vi "FPGA_Clock.vi"(0 "Pause":u8=20, 1 "Data":u32=128, 2 "State":T1) -> ()   [LabVIEW 2015]
uses:
  States.ctl
  <vilib>/rvi/Emulation/niFpgaGetClockAttributes.vi
  <vilib>/rvi/Emulation/niFpgaSctlEmulationGetInTimedLoop.vi
  <vilib>/rvi/Emulation/niFpgaEmulationReportErrorSimple.vi
  <vilib>/rvi/eio/common/nirviEmuTemplateMethod_errors.vi
  <vilib>/rvi/Emulation/niFpgaCriticalErrorInLSC.vi
  <vilib>/eio/EIONode/EIONode.xnode
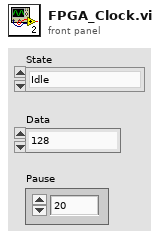
[diagram p1: front panel]
types:
  T1 = typedef "States.ctl" = enum16{"Idle", "CS", "Ready", "Clock High", "Clock Low", "Wait", "Exit"}
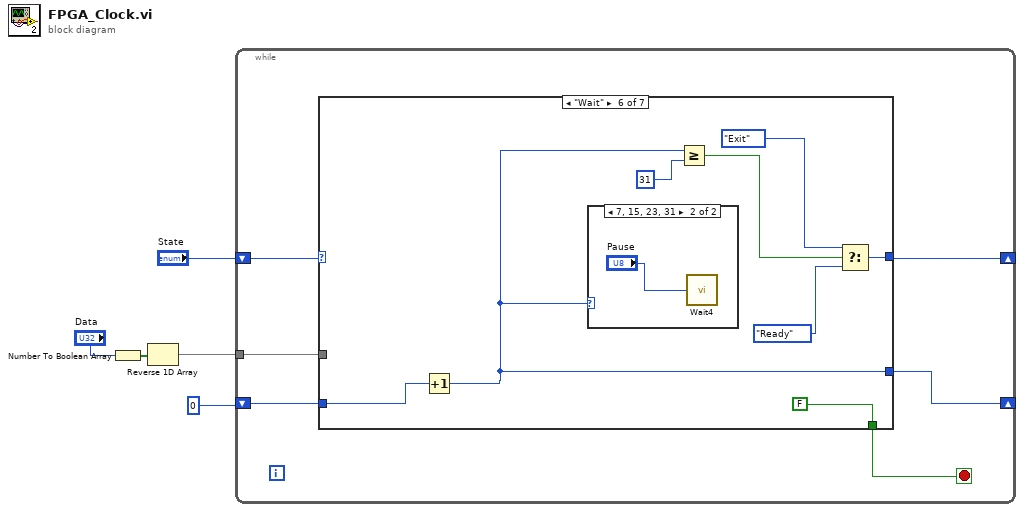
[diagram p0: block diagram]
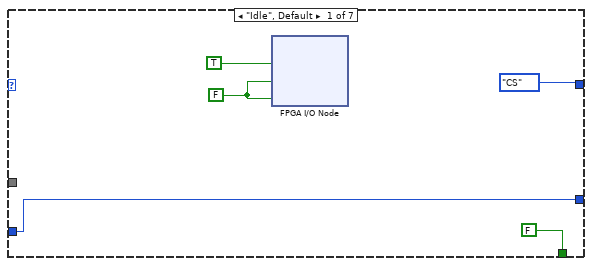
[diagram p2: hidden frame]
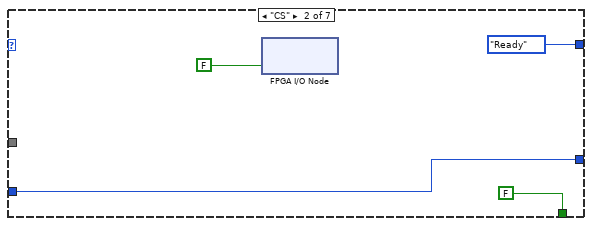
[diagram p3: hidden frame]
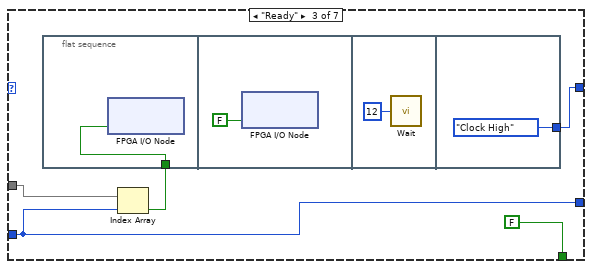
[diagram p4: hidden frame]
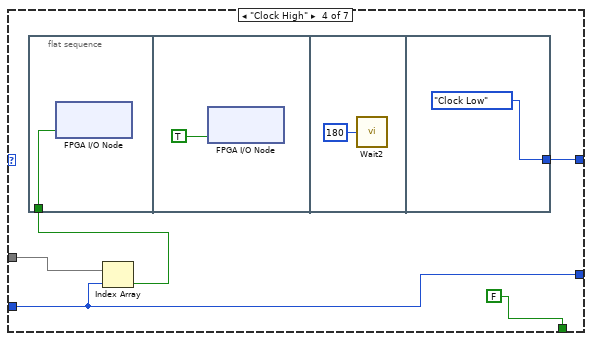
[diagram p5: hidden frame]
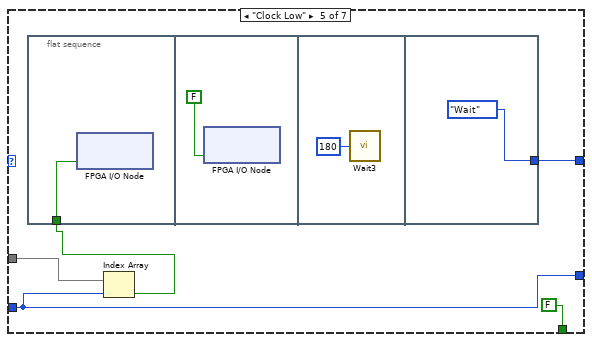
[diagram p6: hidden frame]
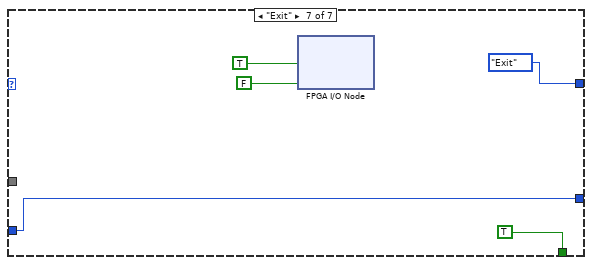
[diagram p8: hidden frame]
diagram:
  n1 = Number To Boolean Array(number="Data") -> (Boolean array=w4:bool[])
  n2 = Reverse 1D Array(array=w4) -> (reversed array=w2:bool[])
  n3 = while {
    shift-right: [w9] -> _
    shift-left: "State" -> [w10]
    tunnel: w2 -> [w8]
    shift-right: [w6] -> _
    shift-left: i16 0 -> [w7]
    stop <- w11 stop-if-true
    n4 = case shown="\"Wait\"" w10 {
      tunnel: [FALSE FALSE FALSE FALSE FALSE FALSE TRUE] -> w11
      tunnel: [States."CS" ("State") States."Ready" ("State") w21 w31 w39 w51 States."Exit" ("State")] -> w9
      tunnel: w8 -> [_ _ w24 w33 w42 _ _]
      tunnel: w7 -> [w13 w17 w23 w32 w41 w49 w58]
      tunnel: [w13 w17 w23 w32 w41 w48 w58] -> w6
      frame "Idle", Default {
        w12 = FALSE
        n5 = xnode "FPGA I/O Node"("CS"=TRUE, "SCLK"=w12, "MOSI"=w12) -> ()  [unwired: 3 in, 3 out]
      }
      frame "CS" {
        n6 = xnode "FPGA I/O Node"("CS"=FALSE) -> ()  [unwired: 1 in, 1 out]
      }
      frame "Ready" {
        n7 = flat-sequence {
          tunnel: w22 -> [w26]
          tunnel: [States."Clock High" ("State")] -> w21
          frame #0 {
            n8 = xnode "FPGA I/O Node"("MOSI"=w26) -> ()  [unwired: 1 in, 1 out]
          }
          frame #1 {
            n9 = xnode "FPGA I/O Node"("SCLK"=FALSE) -> ()  [unwired: 1 in, 1 out]
          }
          frame #2 {
            n10 = call "Wait"("Count(Ticks)"=u8 12) -> ()  [unwired: 1 out]
          }
          frame #3 {
          }
        }
        n11 = Index Array(array=w24, index=w23) -> (element=w22:bool)
      }
      frame "Clock High" {
        n12 = flat-sequence {
          tunnel: w30 -> [w35]
          tunnel: [States."Clock Low" ("State")] -> w31
          frame #0 {
            n13 = xnode "FPGA I/O Node"("MOSI"=w35) -> ()  [unwired: 1 in, 1 out]
          }
          frame #1 {
            n14 = xnode "FPGA I/O Node"("SCLK"=TRUE) -> ()  [unwired: 1 in, 1 out]
          }
          frame #2 {
            n15 = call "Wait2"("Count(Ticks)"=u8 180) -> ()  [unwired: 1 out]
          }
          frame #3 {
          }
        }
        n16 = Index Array(array=w33, index=w32) -> (element=w30:bool)
      }
      frame "Clock Low" {
        n17 = flat-sequence {
          tunnel: w40 -> [w44]
          tunnel: [States."Wait" ("State")] -> w39
          frame #0 {
            n18 = xnode "FPGA I/O Node"("MOSI"=w44) -> ()  [unwired: 1 in, 1 out]
          }
          frame #1 {
            n19 = xnode "FPGA I/O Node"("SCLK"=FALSE) -> ()  [unwired: 1 in, 1 out]
          }
          frame #2 {
            n20 = call "Wait3"("Count(Ticks)"=u8 180) -> ()  [unwired: 1 out]
          }
          frame #3 {
          }
        }
        n21 = Index Array(array=w42, index=w41) -> (element=w40:bool)
      }
      frame "Wait" {
        n22 = Increment(x=w49) -> (x+1=w48:i16)
        n23 = case shown="7, 15, 23, 31" w48 {
          frame 0, Default {
          }
          frame 7, 15, 23, 31 {
            n24 = call "Wait4"("Count(uSec)"="Pause") -> ()  [unwired: 1 out]
          }
        }
        n25 = Greater Or Equal?(x=w48, y=31 ("x")) -> (x >= y?=w54:bool)
        n26 = Select(t=States."Exit" ("State"), s=w54, f=States."Ready" ("State")) -> (s? t:f=w51:T1)
      }
      frame "Exit" {
        n27 = xnode "FPGA I/O Node"("CS"=TRUE, "SCLK"=FALSE) -> ()  [unwired: 2 in, 2 out]
      }
    }
  }
